vi "readTimestampByte.vi"(8 "error in (no error)":errorcluster, 10 "Instruction":u16, 11 "ModbusBuffer in":refnum<class "ModbusBuffer.lvclass">) -> (0 "error out":errorcluster, 2 "Output":u8, 3 "ModbusBuffer out":refnum<class "ModbusBuffer.lvclass">)   [LabVIEW 2016, in "RTModbus.lvlib" / "ModbusBuffer.lvclass"]
uses:
  ModbusBuffer.lvclass
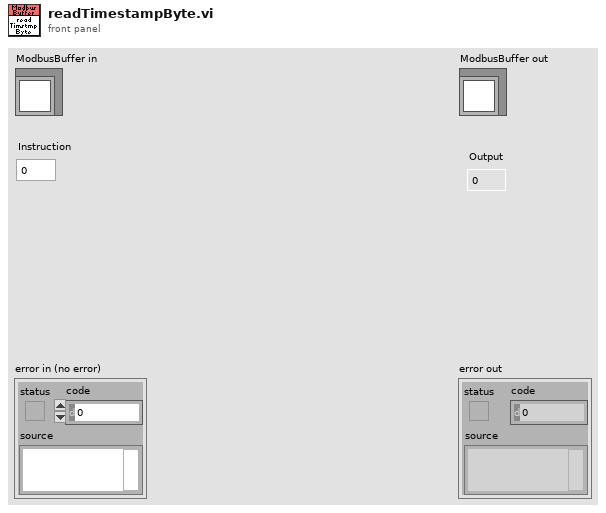
[diagram p1: front panel]
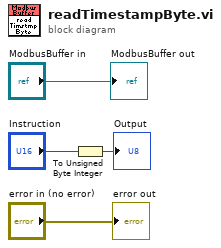
[diagram p0: block diagram]
diagram:
  n1 = To Unsigned Byte Integer(number="Instruction") -> (unsigned 8bit integer=→"Output":u8)
  "error out" <- "error in (no error)"
  "ModbusBuffer out" <- "ModbusBuffer in"
